vi "Write Connections.vi"(5 "Connections":T1[](array[typedef]), 9 "Wire in":refnum<class "Wire.lvclass">) -> (3 "Wire out":refnum<class "Wire.lvclass">)   [LabVIEW 2014, in "Wire.lvclass"]
uses:
  Wire.lvclass
  ConnectionsTD.ctl
  Terminal/Terminal.lvclass
  Wire.lvclass/Wire.ctl
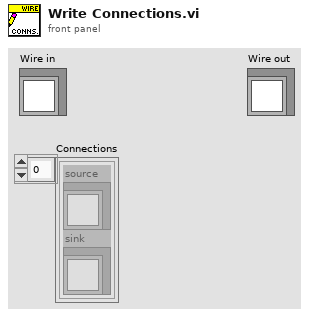
[diagram p1: front panel]
types:
  T1 = typedef "ConnectionsTD.ctl" = cluster{"source":refnum<class "Terminal.lvclass">, "sink":refnum<class "Terminal.lvclass">}
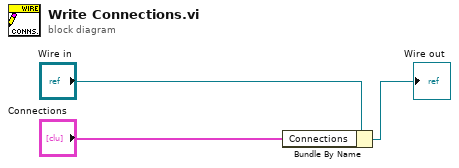
[diagram p0: block diagram]
diagram:
  n1 = Bundle By Name(cluster="Wire in", "Connections"="Connections") -> (→"Wire out":refnum<class "Wire.lvclass">)
